vi "HB_OpenLog.vi"(6 "set time":bool=TRUE, 8 "error in (no error)":errorcluster, 10 "File Name":string, 11 "HBDeviceRef":T1) -> (0 "error out":errorcluster, 3 "HBDeviceRef":T1)   [LabVIEW 2016]
doc: "Opens an existing or creates a new file on the SD card installed in the Huskie Board with the specified file name. The file name must conform to 8.3 FAT file naming conventions.\n\nOnly one file may be opened at a time. If a file is currently opened, it is closed and then the specified file is opened or created. If the file name is too long, it is truncated."
uses:
  <vilib>/Rock Robotics/WPI/SerialPort/WPI_SerialPortRef.ctl
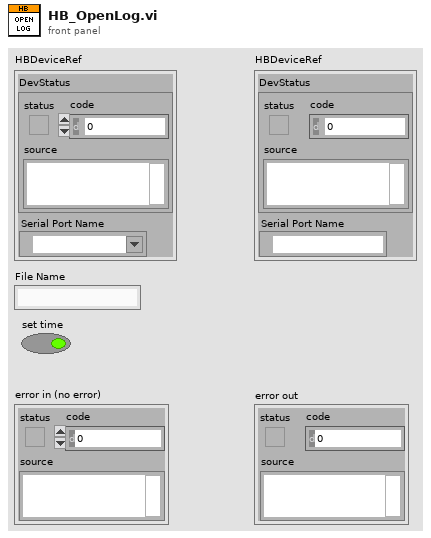
[diagram p1: front panel]
types:
  T1 = typedef "WPI_SerialPortRef.ctl" = cluster{"DevStatus":errorcluster, "Serial Port Name":refnum<visa-resource-name>}
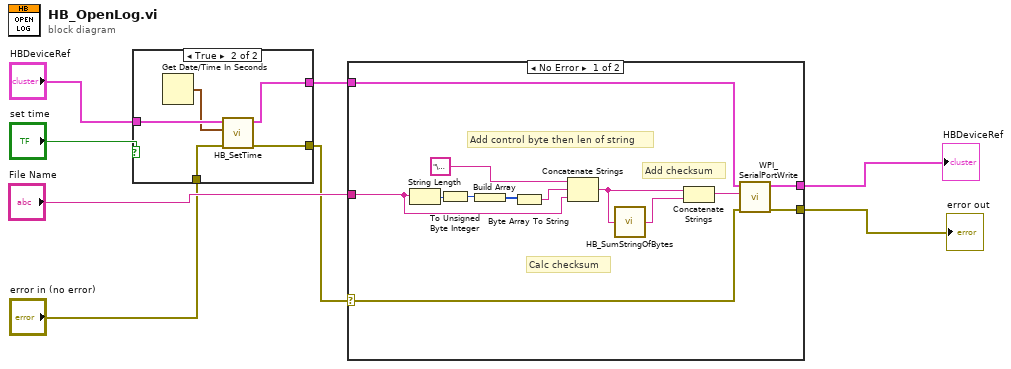
[diagram p0: block diagram]
diagram:
  n1 = case shown="True" "set time" {
    tunnel: "HBDeviceRef" -> [w10 w15]
    tunnel: [w10 w14] -> w4
    tunnel: "error in (no error)" -> [w9 w13]
    tunnel: [w9 w12] -> w2
    frame False {
    }
    frame True {
      n2 = Get Date/Time In Seconds() -> (seconds since 1Jan1904=w11:timestamp)
      n3 = call "HB_SetTime.vi"("error in (no error)"=w13, "Time Stamp"=w11, "HBDeviceRef"=w15) -> ("error IO"=w12:errorcluster, "HBDeviceRef"=w14:T1)  [unwired: 7 in]
    }
  }
  n4 = case shown="No Error" w2 {
    selector: w2 -> [w16 w29]
    tunnel: "File Name" -> [w22 _]
    tunnel: w4 -> [w21 w30]
    tunnel: [w20 w30] -> w7
    tunnel: [w19 w29] -> w6
    frame No Error {
      # "Calc checksum"
      # "Add checksum"
      # "Add control byte then len of string"
      n5 = String Length(string=w22) -> (length=w24:i32)
      n6 = To Unsigned Byte Integer(number=w24) -> (unsigned 8bit integer=w27:u8)
      n7 = Build Array(w27) -> (w26:u8[])
      n8 = Byte Array To String(unsigned byte array=w26) -> (string=w25:string)
      n9 = Concatenate Strings("\u0003", w25, w22) -> (w18:string)
      n10 = call "HB_SumStringOfBytes.vi"("String Of Bytes"=w18) -> ("Sum as String"=w17:string)
      n11 = Concatenate Strings(w18, w17) -> (w23:string)
      n12 = call <vilib>:"WPI_SerialPortWrite.vi"("error in (no error)"=w16, "Buffer"=w23, "SerialPortRef"=w21) -> ("error out"=w19:errorcluster, "SerialPortRef"=w20:T1)  [unwired: 6 in, 1 out]
    }
    frame Error {
    }
  }
  "HBDeviceRef" <- w7
  "error out" <- w6
